vi "Destroy.vi"(8 "Error In":errorcluster, 11 "Object in":refnum<class "WebView.Tabulator.lvclass">) -> (0 "Error Out":errorcluster)   [LabVIEW 2024, in "WebView.Tabulator.lvclass"]
uses:
  WebView.Tabulator.lvclass
  WebView.Tabulator.lvclass/WebView.Tabulator.ctl
  WebView_class/WebView.lvclass
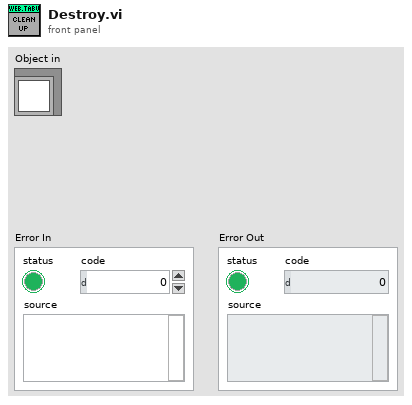
[diagram p1: front panel]
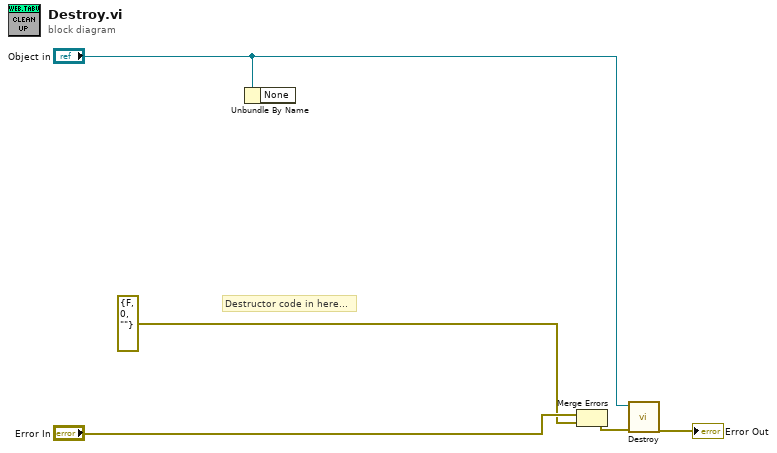
[diagram p0: block diagram]
diagram:
  # "Destructor code in here..."
  n1 = Unbundle By Name("Object in") -> ()  [unwired: 1 out]
  n2 = Merge Errors("Error In", errorcluster {"status"=FALSE, "code"=0, "source"=""} ("error in (no error)")) -> (w2:errorcluster)
  n3 = call-parent "Destroy.vi"("Error In"=w2, "WebView in"="Object in") -> ("Error Out"=→"Error Out":errorcluster)  [unwired: 9 in]
